vi "Save-configuration.vi"(8 "error in (no error)":errorcluster, 11 "Object ref in":T1) -> (0 "error out":errorcluster, 1 "Succes?":bool, 3 "Object ref out":T1)   [LabVIEW 2013, in "SLMControl.lvlib" / "SC-Main.lvclass"]
uses:
  SC-Main.lvclass
  Object-reference.ctl
  SC-Main.lvclass/SC-Main.ctl
  Configuration-data.ctl
  Read Status.vi
  Read Deposition files.vi
  Read Lasing files.vi
  <vilib>/Utility/xml.llb/Write to XML File(string).vi
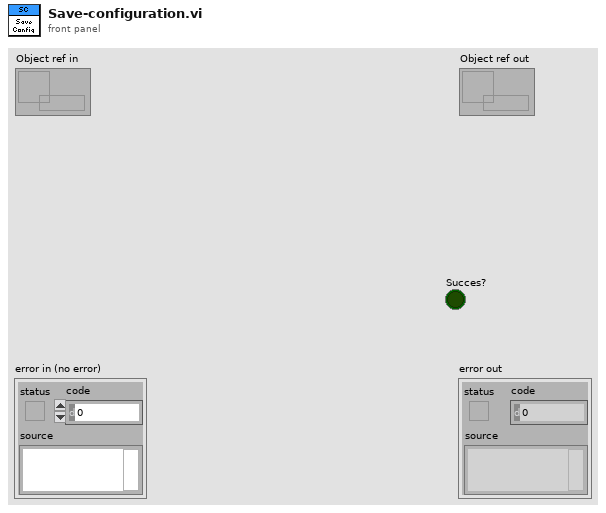
[diagram p1: front panel]
types:
  T1 = typedef "SLMControl.lvlib/SC-Main.lvclass/Object-reference.ctl" = refnum<data-value>
  T2 = typedef "SLMControl.lvlib/SC-Main.lvclass/Configuration-data.ctl" = cluster{"Deposition files":path[], "Lasing files":path[]}
  T3 = typedef "SLMControl.lvlib/SC-Main.lvclass/Client-status.ctl" = enum16{"Idle", "Initialized", "Configured", "Activated", "Started", "Paused", "Stopped", "Reset", "Error", "Exited"}
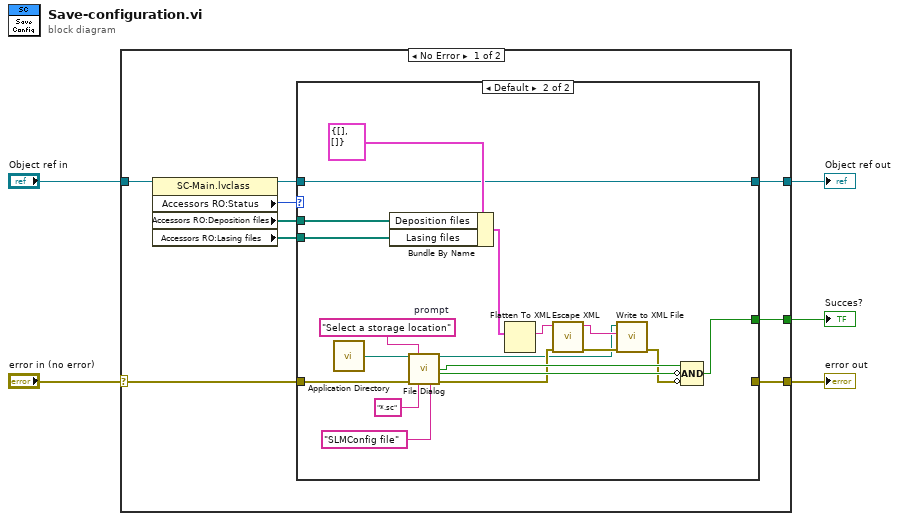
[diagram p0: block diagram]
diagram:
  n1 = case shown="No Error" "error in (no error)" {
    selector: "error in (no error)" -> [w14 w37]
    tunnel: [w11 w37] -> w4
    tunnel: [w10 w36] -> w2
    tunnel: "Object ref in" -> [w13 w36]
    tunnel: [w6 _] -> w1
    frame No Error {
      n2 = property class="SC-Main.lvclass"(reference=w13) -> (reference out=w12:T1, "Accessors RO:Status"=w9:T3, "Accessors RO:Deposition files"=w8:path[], "Accessors RO:Lasing files"=w7:path[])  [unwired: 1 in, 1 out]
      n3 = case shown="Default" w9 {
        tunnel: w14 -> [w16 w32]
        tunnel: w12 -> [w15 w18]
        tunnel: [w16 _] -> w11
        tunnel: [w15 w18] -> w10
        tunnel: w8 -> [_ w28]
        tunnel: w7 -> [_ w27]
        tunnel: [_ w17] -> w6
        frame "Error" {
        }
        frame Default {
          w34 = "Select a storage location"  # prompt
          n4 = call <vilib>:"Application Directory.vi"() -> ("Application Directory"=w35:path)
          n5 = Bundle By Name(cluster=T2 {"Deposition files"=[], "Lasing files"=[]} ("Configuration data"), "Deposition files"=w28, "Lasing files"=w27) -> (w22:T2)
          n6 = call "File Dialog"("start path"=w35, "prompt"=w34, "error in"=w32, "pattern (all files)"="*.sc", "pattern label"="SLMConfig file") -> ("selected path"=w19:path, "exists"=w30:bool, "cancelled"=w29:bool, "error out"=w21:errorcluster)  [unwired: 7 in]
          n7 = Flatten To XML(anything=w22) -> (xml string=w25:string)
          n8 = call <vilib>:"Escape XML.vi"("error in (no error)"=w21, "XML String In"=w25) -> ("error out"=w24:errorcluster, "XML String Out"=w23:string)  [unwired: 8 in]
          n9 = call-poly <vilib>:"Write to XML File.vi"("error in (no error)"=w24, "XML Input"=w23, "XML File Path"=w19) -> ("error out"=w20:errorcluster)  [unwired: 6 in, 2 out]
          n10 = Compound Arithmetic op=AND(w30, invert w29, invert w20) -> (w17:bool)
        }
      }
    }
    frame Error {
    }
  }
  "error out" <- w4
  "Object ref out" <- w2
  "Succes?" <- w1
